vi "FindLaserDot.vi"(11 "Image Input":T1=refnum) -> (0 "Y Location":i32, 1 "X Location":i32, 2 "Max Pixel Value":i32, 3 "Array of Pixel Value, X Location, Y Location":i32[][](array[numeric])=[[47, 47, 47, 47, 47, 47, 47, 47, 47, 48, 47, 47, 47, 47, 47, 47, 47, 47, 48, 47, 47, 48, 47, 47, 47, 47, 48, 48, 47, 47, 47, 48, 48, 47, 47, 47, 47, 48, 48, 48, 48, 47, 48, 47, 47, 48, 48, 48, 48, 48, 48, 48, 48, 48, 48, 48, 48, 48, 47, 47, 49, 48, 48, 48, 48, 47, 48, 48, 48, 48, 48, 49, 47, 48, 48, 48, 48, 48, 48, 48, 48, 49, 48, 48, 49, 49, 48, 48, 48, 49, 50, 48, 49, 49, 48, 48, 48, 48, 49, 48, 48, 48, 48, 49, 49, 49, 49, 49, 49, 49, 48, 49, 49, 49, 48, 49, 49, 49, 49, 49, 48, 49, 49, 49, 48, 49, 49, 49, 49, 49, 49, 49, 50, 49, 49, 49, 49, 49, 49, 49, 49, 49, 49, 50, 49, 50, 49, 49, 49, 50, 49, 50, 49, 50, 49, 49, 50, 50, 49, 50, 50, 49, 50, 49, 49, 50, 50, 49, 50, 50, 50, 50, 50, 50, 50, 50, 50, 50, 49, 50, 50, 50, 50, 50, 49, 50, 50, 50, 49, 49, 50, 50, 50, 50, 50, 50, 50, 50, 50, 50, 50, 50, 50, 50, 50, 51, 50, 50, 51, 50, 50, 51, 51, 51, 51, 50, 51, 50, 51, 51, 51, 51, 50, 51, 50, 51, 51, 51, 50, 51, 51, 51, 51, 51, 51, 50, 51, 51, 51, 51, 52, 51, 51, 51, 51, 51, 51, 51, 51, 51, 51, 52, 51, 51, 51, 51, 51, 51, 51, 51, 51, 52, 52, 51, 51, 51, 51, 51, 51, 51, 51, 51, 52, 52, 51, 52, 51, 51, 51, 52, 51, 52, 52, 52, 52, 52, 53, 52, 53, 51, 52, 52, 52, 52, 52, 52, 52, 52, 52, 52, 54, 53, 52, 52, 52, 53, 52, 52, 53, 52, 52, 52, 53, 52, 53, 53, 52, 52, 52, 53, 52, 53, 52, 52, 53, 53, 52, 53, 53, 53, 53, 53, 53, 53, 53, 53, 53, 53, 53, 53, 53, 54, 53, 53, 54, 53, 53, 53, 53, 54, 53, 54, 54, 53, 53, 54, 54, 53, 53, 54, 54, 55, 54, 54, 53, 54, 54, 54, 54, 54, 54, 54, 55, 54, 55, 55, 54, 54, 54, 54, 54, 54, 54, 55, 54, 55, 54, 55, 55, 55, 55, 55, 55, 55, 55, 55, 56, 55, 55, 55, 55, 55, 55, 55, 55, 55, 56, 55, 55, 55, 56, 56, 56, 55, 55, 55, 56, 55, 56, 56, 56, 56, 55, 56, 55, 56, 56, 56, 56, 56, 56, 57, 56, 56, 56, 56, 57, 56, 56, 57, 56, 56, 57, 57, 56, 57, 56, 56, 56, 57], [50, 51, 52, 53, 54, 55, 56, 57, 58, 59, 60, 61, 62, 63, 64, 65, 66, 67, 68, 69, 70, 71, 72, 73, 74, 75, 76, 77, 78, 79, 80, 81, 82, 83, 84, 85, 86, 87, 88, 89, 90, 91, 92, 93, 94, 95, 96, 97, 98, 99, 100, 101, 102, 103, 104, 105, 106, 107, 108, 109, 110, 111, 112, 113, 114, 115, 116, 117, 118, 119, 120, 121, 122, 123, 124, 125, 126, 127, 128, 129, 130, 131, 132, 133, 134, 135, 136, 137, 138, 139, 140, 141, 142, 143, 144, 145, 146, 147, 148, 149, 150, 151, 152, 153, 154, 155, 156, 157, 158, 159, 160, 161, 162, 163, 164, 165, 166, 167, 168, 169, 170, 171, 172, 173, 174, 175, 176, 177, 178, 179, 180, 181, 182, 183, 184, 185, 186, 187, 188, 189, 190, 191, 192, 193, 194, 195, 196, 197, 198, 199, 200, 201, 202, 203, 204, 205, 206, 207, 208, 209, 210, 211, 212, 213, 214, 215, 216, 217, 218, 219, 220, 221, 222, 223, 224, 225, 226, 227, 228, 229, 230, 231, 232, 233, 234, 235, 236, 237, 238, 239, 240, 241, 242, 243, 244, 245, 246, 247, 248, 249, 250, 251, 252, 253, 254, 255, 256, 257, 258, 259, 260, 261, 262, 263, 264, 265, 266, 267, 268, 269, 270, 271, 272, 273, 274, 275, 276, 277, 278, 279, 280, 281, 282, 283, 284, 285, 286, 287, 288, 289, 290, 291, 292, 293, 294, 295, 296, 297, 298, 299, 300, 301, 302, 303, 304, 305, 306, 307, 308, 309, 310, 311, 312, 313, 314, 315, 316, 317, 318, 319, 320, 321, 322, 323, 324, 325, 326, 327, 328, 329, 330, 331, 332, 333, 334, 335, 336, 337, 338, 339, 340, 341, 342, 343, 344, 345, 346, 347, 348, 349, 350, 351, 352, 353, 354, 355, 356, 357, 358, 359, 360, 361, 362, 363, 364, 365, 366, 367, 368, 369, 370, 371, 372, 373, 374, 375, 376, 377, 378, 379, 380, 381, 382, 383, 384, 385, 386, 387, 388, 389, 390, 391, 392, 393, 394, 395, 396, 397, 398, 399, 400, 401, 402, 403, 404, 405, 406, 407, 408, 409, 410, 411, 412, 413, 414, 415, 416, 417, 418, 419, 420, 421, 422, 423, 424, 425, 426, 427, 428, 429, 430, 431, 432, 433, 434, 435, 436, 437, 438, 439, 440, 441, 442, 443, 444, 445, 446, 447, 448, 449, 450, 451, 452, 453, 454, 455, 456, 457, 458, 459, 460, 461, 462, 463, 464, 465, 466, 467, 468, 469, 470, 471, 472, 473, 474, 475, 476, 477, 478, 479, 480, 481, 482, 483, 484, 485, 486, 487, 488, 489, 490, 491, 492, 493, 494, 495, 496, 497, 498, 499], [156, 185, 250, 221, 268, 284, 226, 177, 121, 158, 183, 134, 311, 231, 179, 239, 153, 126, 230, 209, 300, 300, 224, 211, 180, 173, 314, 408, 257, 237, 254, 455, 200, 293, 169, 201, 235, 204, 335, 267, 310, 292, 306, 160, 235, 313, 410, 422, 417, 252, 376, 317, 341, 362, 262, 379, 336, 266, 168, 205, 392, 278, 277, 299, 385, 165, 312, 263, 324, 202, 204, 387, 171, 239, 312, 300, 384, 328, 331, 274, 311, 326, 181, 181, 328, 468, 242, 259, 255, 335, 254, 253, 326, 312, 242, 248, 270, 221, 315, 229, 283, 184, 185, 361, 260, 358, 253, 278, 379, 250, 162, 269, 334, 268, 267, 279, 399, 275, 330, 305, 177, 295, 294, 427, 97, 334, 293, 285, 235, 269, 344, 294, 294, 235, 263, 290, 218, 311, 197, 254, 356, 288, 281, 499, 314, 202, 282, 359, 168, 433, 231, 281, 181, 409, 207, 202, 422, 222, 230, 228, 403, 206, 430, 202, 195, 238, 238, 159, 302, 322, 321, 454, 396, 263, 285, 383, 409, 377, 220, 351, 335, 403, 358, 279, 242, 275, 248, 334, 106, 201, 262, 446, 358, 222, 297, 303, 197, 277, 320, 253, 341, 196, 294, 284, 244, 385, 369, 298, 385, 295, 198, 408, 407, 407, 282, 258, 443, 268, 325, 332, 324, 377, 222, 368, 306, 324, 364, 330, 198, 337, 321, 344, 282, 351, 350, 223, 452, 336, 343, 345, 350, 335, 210, 219, 302, 212, 235, 212, 315, 284, 312, 320, 272, 294, 240, 184, 246, 247, 248, 329, 270, 304, 275, 269, 243, 270, 208, 287, 194, 278, 245, 228, 307, 327, 173, 251, 175, 178, 173, 281, 156, 386, 301, 352, 384, 301, 414, 384, 383, 186, 360, 326, 338, 325, 302, 329, 303, 340, 339, 331, 407, 407, 311, 400, 292, 341, 377, 365, 430, 357, 222, 382, 378, 277, 368, 378, 253, 270, 277, 400, 258, 422, 128, 257, 268, 262, 261, 328, 393, 302, 353, 385, 259, 260, 280, 281, 259, 190, 396, 286, 310, 320, 194, 270, 474, 378, 245, 244, 160, 432, 306, 383, 395, 243, 246, 274, 311, 176, 175, 401, 288, 304, 318, 292, 148, 317, 318, 334, 248, 304, 287, 350, 452, 309, 388, 388, 256, 160, 301, 442, 212, 210, 257, 364, 236, 236, 237, 204, 425, 281, 338, 278, 294, 462, 288, 293, 294, 285, 271, 272, 272, 264, 309, 488, 272, 251, 421, 171, 261, 261, 351, 380, 418, 428, 329, 221, 330, 222, 228, 215, 435, 444, 227, 311, 184, 234, 234, 281, 298, 282, 282, 282, 191, 190, 219, 212, 361, 209, 221, 335, 284, 203, 198, 199, 67, 307, 159, 159, 223, 224]])   [LabVIEW 2015]
uses:
  <vilib>/vision/Image Controls.llb/IMAQ Image.ctl
panel:
  out "image display":T1(plugin-control)
  in  "Y Max":i32=1180
  in  "X Max":i32=1900
  in  "Y Minimum":i32=20
  in  "X Minimum":i32=20
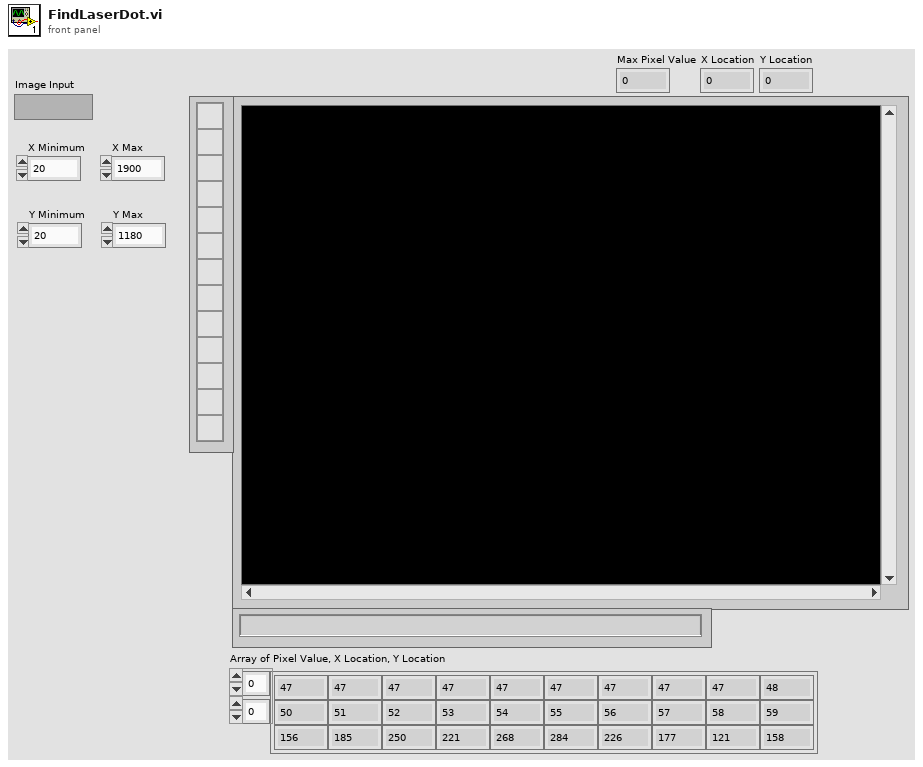
[diagram p1: front panel]
types:
  T1 = typedef "IMAQ Image.ctl" = refnum<image>
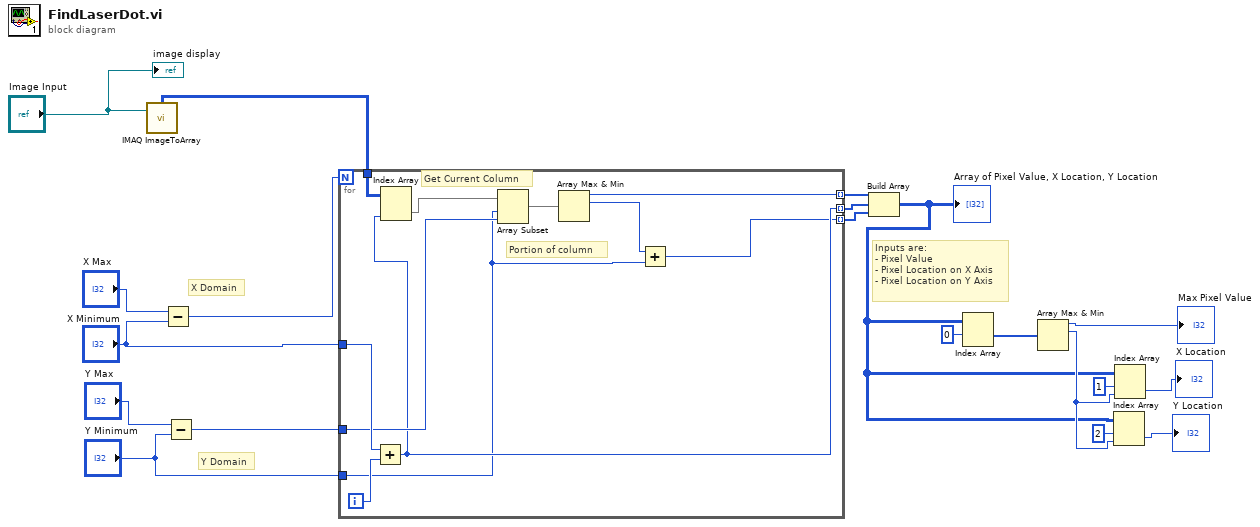
[diagram p0: block diagram]
diagram:
  # "Inputs are:\n- Pixel Value\n- Pixel Location on X Axis\n- Pixel Location on Y Axis"
  # "Y Domain"
  # "X Domain"
  n1 = call "IMAQ ImageToArray"("Image"="Image Input") -> ("Image Pixels (U8)"=w19:u8[][])  [unwired: 2 in, 5 out]
  n2 = Subtract(x="X Max", y="X Minimum") -> (x-y=w20:i32)
  n3 = Subtract(x="Y Max", y="Y Minimum") -> (x-y=w18:i32)
  n4 = for {
    N: w20 -> [_]
    tunnel: "X Minimum" -> [w30]
    tunnel: w19 -> [w29]
    tunnel: "Y Minimum" -> [w22]
    tunnel: w18 -> [w27]
    tunnel: [w25] -> w17 mode=indexing
    tunnel: [w24] -> w16 mode=indexing
    tunnel: [w21] -> w15 mode=indexing
    i -> [w31]
    # "Portion of column"
    # "Get Current Column"
    n5 = Add(x=w30, y=w31) -> (x+y=w24:i32)
    n6 = Index Array(array=w29, index (col)=w24) -> (element=w28:u8[])  [unwired: 1 in]
    n7 = Array Subset(array=w28, index=w22, length=w27) -> (w26:u8[])
    n8 = Array Max & Min(array=w26) -> (max value=w25:u8, max index (indices)=w23:i32)  [unwired: 2 out]
    n9 = Add(x=w23, y=w22) -> (x+y=w21:i32)
  }
  n10 = Build Array(w17, w16, w15) -> (w4:i32[][])
  "Array of Pixel Value, X Location, Y Location" <- w4
  n11 = Index Array(array=w4, index (row)=0) -> (element=w8:i32[])  [unwired: 1 in]
  n12 = Array Max & Min(array=w8) -> (max value=→"Max Pixel Value":i32, max index (indices)=w5:i32)  [unwired: 2 out]
  n13 = Index Array(array=w4, index (row)=2 ("disabled index (row)"), index (col)=w5) -> (element=→"Y Location":i32)
  n14 = Index Array(array=w4, index (row)=1 ("disabled index (row)"), index (col)=w5) -> (element=→"X Location":i32)
  "image display" <- "Image Input"
